vi "three_color_2D_AFM_synched.vi"() -> ()   [LabVIEW 2017]
uses:
  <vilib>/DAQmx/write.llb/DAQmx Write (Analog DBL 1Chan 1Samp).vi
  <vilib>/DAQmx/write.llb/DAQmx Write (Analog 2D DBL NChan NSamp).vi
  <vilib>/DAQmx/create/channels.llb/DAQmx Create Channel (AO-Voltage-Basic).vi
  <vilib>/DAQmx/miscellaneous.llb/DAQmx Fill In Error Info.vi
  <vilib>/DAQmx/configure/timing.llb/DAQmx Timing (Sample Clock).vi
  <vilib>/DAQmx/configure/trigger.llb/DAQmx Start Trigger (Digital Edge).vi
  <vilib>/DAQmx/write.llb/DAQmx Write (Analog 1D DBL NChan 1Samp).vi
  <resource>/objmgr/daqmx.rc
panel:
  in  "Listbox 3":i32(listbox)=3
  in  "Laser 3 (0-10v)":dbl=3.0
  out "Focal Distance (um)":dbl
  out "Diopter":dbl
  in  "ETL3 (v) [4.76V allows light passing through unaltered]":dbl(slide)=4.76 min=-10.0 max=10.0 step=0.01 scale=-10.0..10.0
  in  "Y multiplier":dbl=1.0
  in  "X multiplier":dbl=-1.0
  in  "Y (v)":dbl(slide) min=-10.0 max=10.0 step=0.01 scale=-10.0..10.0
  in  "X (v)":dbl(slide) min=-10.0 max=10.0 step=0.01 scale=-10.0..10.0
  in  "Combined Movement (v)\nEquation: X * X Multiplier + Y * Y Multiplier":dbl(slide) min=-10.0 max=10.0 step=0.01 scale=-10.0..10.0
  out "Expected AFM Frequency (HZ)":dbl
  in  "Listbox 2":i32(listbox)=3
  in  "Listbox":i32(listbox)=1
  in  "Laser 2 (0-10v)":dbl=3.0
  in  "Laser 1 (0-10v)":dbl=3.0
  in  "OFF Time(ms)":dbl=100.0
  in  "ON Time(ms)":dbl=300.0
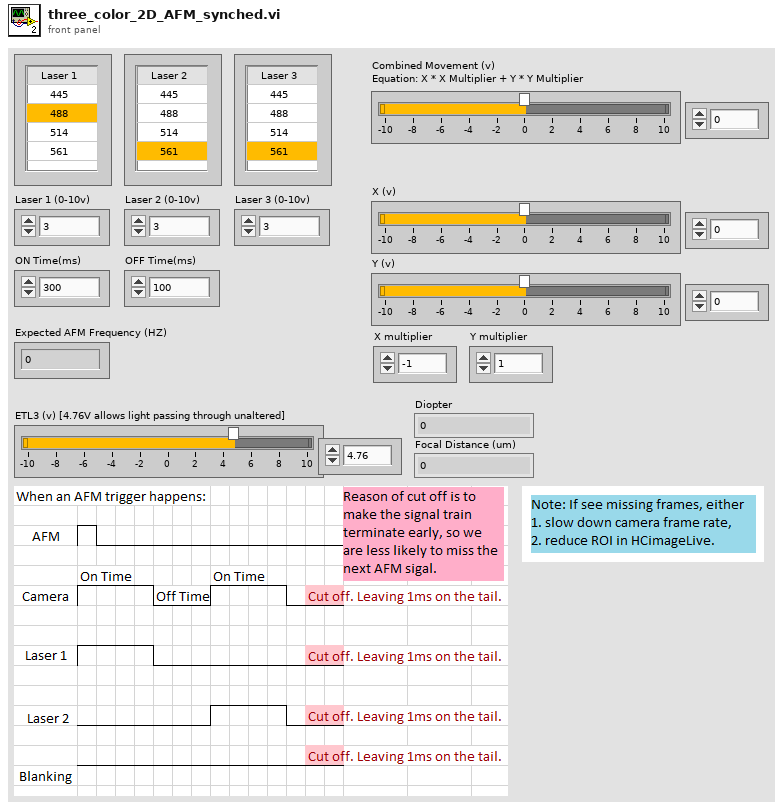
[diagram p1: front panel]
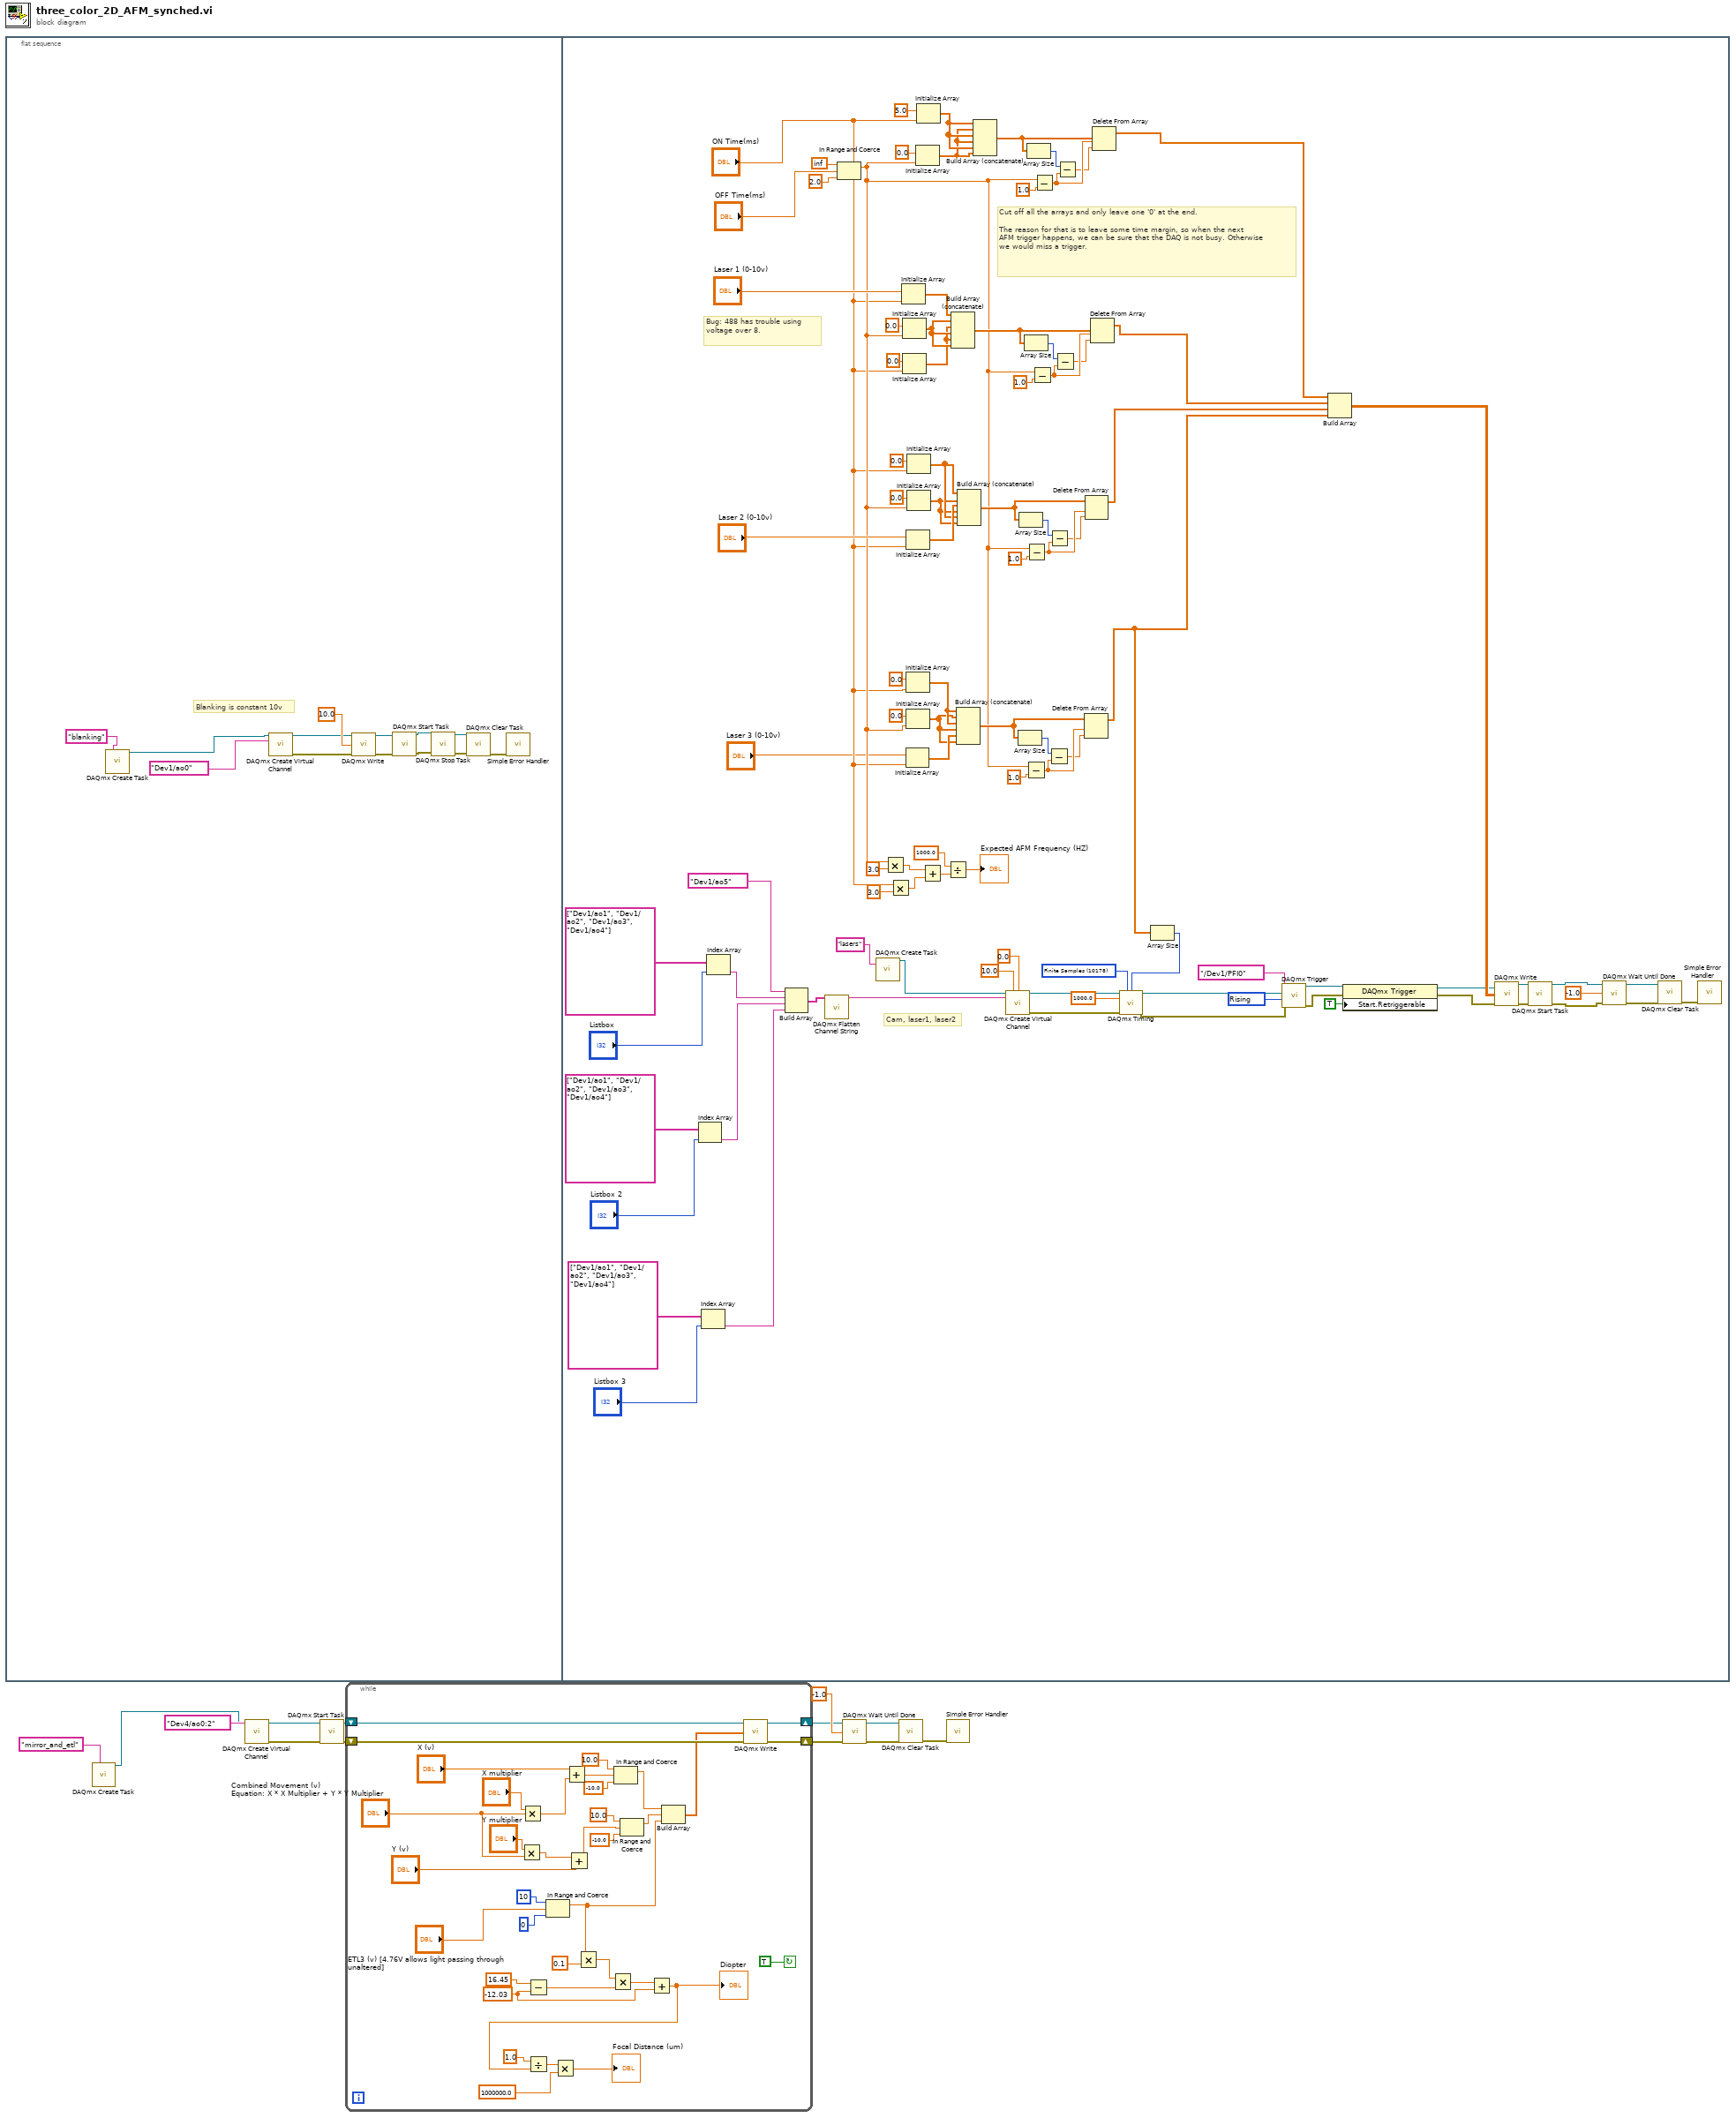
[diagram p0: block diagram]
diagram:
  n1 = flat-sequence {
    frame #0 {
      # "Blanking is constant 10v"
      n2 = call <vilib>:"DAQmx Create Task.vi"("new task name"="blanking" ("name to assign")) -> ("task out"=w16:refnum<k21>)  [unwired: 13 in, 1 out]
      n3 = call-poly <vilib>:"DAQmx Create Virtual Channel.vi"("task in"=w16, "physical channels"=tag "Dev1/ao0") -> ("task out"=w24:refnum<k21>, "error out"=w23:errorcluster)  [unwired: 12 in]
      n4 = call-poly <vilib>:"DAQmx Write.vi"("task/channels in"=w24, "data"=10.0, "error in"=w23) -> ("task out"=w22:refnum<k21>, "error out"=w21:errorcluster)  [unwired: 10 in, 1 out]
      n5 = call <vilib>:"DAQmx Start Task.vi"("task/channels in"=w22, "error in"=w21) -> ("task out"=w15:refnum<k21>, "error out"=w14:errorcluster)  [unwired: 12 in]
      n6 = call <vilib>:"DAQmx Stop Task.vi"("task/channels in"=w15, "error in"=w14) -> ("task out"=w20:refnum<k21>, "error out"=w19:errorcluster)  [unwired: 12 in]
      n7 = call <vilib>:"DAQmx Clear Task.vi"("task in"=w20, "error in"=w19) -> ("error out"=w26:errorcluster)  [unwired: 13 in]
      n8 = call <vilib>:"Simple Error Handler.vi"("error in (no error)"=w26) -> ()  [unwired: 4 in, 5 out]
    }
    frame #1 {
      w66 = 10280 items=["Rising"=10280, "Falling"=10171] ("edge")
      w62 = 10178 items=["Finite Samples"=10178, "Continuous Samples"=10123, "Hardware Timed Single Point"=12522] ("sample mode")
      # "Bug: 488 has trouble using voltage over 8."
      # "Cut off all the arrays and only leave one '0' at the end.\n\nThe reason for that is to leave some time margin, so when the next \nAFM trigger happens, we can be sure that the DAQ is not busy. Otherwise\nwe would miss a trigger."
      # "Cam, laser1, laser2"
      n9 = Index Array(array=tag[] ["Dev1/ao1", "Dev1/ao2", "Dev1/ao3", "Dev1/ao4"], index="Listbox 2") -> (element=w117:tag)
      n10 = Index Array(array=tag[] ["Dev1/ao1", "Dev1/ao2", "Dev1/ao3", "Dev1/ao4"], index="Listbox 3") -> (element=w48:tag)
      n11 = Index Array(array=tag[] ["Dev1/ao1", "Dev1/ao2", "Dev1/ao3", "Dev1/ao4"], index="Listbox") -> (element=w116:tag)
      n12 = Build Array(tag "Dev1/ao5" ("physical channels"), w116, w117, w48) -> (w118:tag[])
      n13 = call <vilib>:"DAQmx Flatten Channel String.vi"("names in"=w118) -> ("names out"=w121:string)  [unwired: 13 in, 1 out]
      n14 = In Range and Coerce(upper limit=inf, x="OFF Time(ms)", lower limit=2.0) -> (coerced(x)=w40:dbl)  [unwired: 1 out]
      n15 = call <vilib>:"DAQmx Create Task.vi"("new task name"="lasers" ("name to assign")) -> ("task out"=w123:refnum<k21>)  [unwired: 13 in, 1 out]
      n16 = Multiply(x=w40, y=3.0) -> (x*y=w106:dbl)
      n17 = Multiply(x="ON Time(ms)", y=3.0) -> (x*y=w105:dbl)
      n18 = Initialize Array("Laser 1 (0-10v)", "ON Time(ms)") -> (w80:dbl[])
      n19 = Initialize Array(0.0 ("element"), w40) -> (w33:dbl[])
      n20 = Initialize Array(0.0 ("element"), "ON Time(ms)") -> (w32:dbl[])
      n21 = Initialize Array("Laser 3 (0-10v)", "ON Time(ms)") -> (w28:dbl[])
      n22 = Initialize Array("Laser 2 (0-10v)", "ON Time(ms)") -> (w85:dbl[])
      n23 = Initialize Array(0.0 ("element"), "ON Time(ms)") -> (w29:dbl[])
      n24 = Initialize Array(0.0 ("element"), w40) -> (w27:dbl[])
      n25 = Initialize Array(0.0 ("element"), "ON Time(ms)") -> (w31:dbl[])
      n26 = Initialize Array(0.0 ("element"), w40) -> (w30:dbl[])
      n27 = Initialize Array(0.0 ("element"), w40) -> (w34:dbl[])
      n28 = Initialize Array(5.0 ("element"), "ON Time(ms)") -> (w35:dbl[])
      n29 = Add(x=w106, y=w105) -> (x+y=w107:dbl)
      n30 = Divide(x=1000.0, y=w107) -> (x/y=→"Expected AFM Frequency (HZ)":dbl)
      n31 = Build Array (concatenate)(w80, w33, w32, w33, w32, w33) -> (w84:dbl[])
      n32 = Build Array (concatenate)(w29, w27, w29, w27, w28, w27) -> (w47:dbl[])
      n33 = Build Array (concatenate)(w31, w30, w85, w30, w31, w30) -> (w89:dbl[])
      n34 = Build Array (concatenate)(w35, w34, w35, w34, w35, w34) -> (w76:dbl[])
      n35 = call-poly <vilib>:"DAQmx Create Virtual Channel.vi"("task in"=w123, "maximum value"=10.0, "minimum value"=0.0, "physical channels"=w121) -> ("task out"=w97:refnum<k21>, "error out"=w98:errorcluster)  [unwired: 10 in]
      n36 = Array Size(array=w47) -> (size(s)=w44:i32)
      n37 = Array Size(array=w89) -> (size(s)=w86:i32)
      n38 = Array Size(array=w84) -> (size(s)=w81:i32)
      n39 = Subtract(x=w40, y=1.0) -> (x-y=w46:dbl)
      n40 = Subtract(x=w40, y=1.0) -> (x-y=w88:dbl)
      n41 = Array Size(array=w76) -> (size(s)=w77:i32)
      n42 = Subtract(x=w40, y=1.0) -> (x-y=w83:dbl)
      n43 = Subtract(x=w40, y=1.0) -> (x-y=w79:dbl)
      n44 = Subtract(x=w44, y=w46) -> (x-y=w45:dbl)
      n45 = Subtract(x=w86, y=w88) -> (x-y=w87:dbl)
      n46 = Subtract(x=w81, y=w83) -> (x-y=w82:dbl)
      n47 = Subtract(x=w77, y=w79) -> (x-y=w78:dbl)
      n48 = Delete From Array(array=w47, length=w46, index=w45) -> (array with subset deleted=w36:dbl[])  [unwired: 1 out]
      n49 = Delete From Array(array=w89, length=w88, index=w87) -> (array with subset deleted=w111:dbl[])  [unwired: 1 out]
      n50 = Delete From Array(array=w84, length=w83, index=w82) -> (array with subset deleted=w109:dbl[])  [unwired: 1 out]
      n51 = Delete From Array(array=w76, length=w79, index=w78) -> (array with subset deleted=w108:dbl[])  [unwired: 1 out]
      n52 = Array Size(array=w36) -> (size(s)=w122:i32)
      n53 = call-poly <vilib>:"DAQmx Timing.vi"("task/channels in"=w97, "sample mode"=w62, "samples per channel"=w122, "rate"=1000.0, "error in"=w98) -> ("task out"=w99:refnum<k21>, "error out"=w100:errorcluster)  [unwired: 9 in]
      n54 = call-poly <vilib>:"DAQmx Trigger.vi"("task/channels in"=w99, "source"=tag "/Dev1/PFI0", "edge"=w66, "error in"=w100) -> ("task out"=w101:refnum<k21>, "error out"=w104:errorcluster)  [unwired: 10 in]
      n55 = Build Array(w108, w109, w111, w36) -> (w110:dbl[][])
      n56 = property class="DAQmx Trigger"(reference=w101, error in=w104, "Start.Retriggerable"=TRUE) -> (reference out=w102:refnum<k21>, error out=w103:errorcluster)
      n57 = call-poly <vilib>:"DAQmx Write.vi"("task/channels in"=w102, "data"=w110, "error in"=w103) -> ("task out"=w95:refnum<k21>, "error out"=w96:errorcluster)  [unwired: 10 in, 1 out]
      n58 = call <vilib>:"DAQmx Start Task.vi"("task/channels in"=w95, "error in"=w96) -> ("task out"=w94:refnum<k21>, "error out"=w93:errorcluster)  [unwired: 12 in]
      n59 = call <vilib>:"DAQmx Wait Until Done.vi"("task/channels in"=w94, "timeout (sec)"=-1.0, "error in"=w93) -> ("task out"=w91:refnum<k21>, "error out"=w92:errorcluster)  [unwired: 11 in]
      n60 = call <vilib>:"DAQmx Clear Task.vi"("task in"=w91, "error in"=w92) -> ("error out"=w90:errorcluster)  [unwired: 13 in]
      n61 = call <vilib>:"Simple Error Handler.vi"("error in (no error)"=w90) -> ()  [unwired: 4 in, 5 out]
    }
  }
  n62 = call <vilib>:"DAQmx Create Task.vi"("new task name"="mirror_and_etl" ("name to assign")) -> ("task out"=w1:refnum<k21>)  [unwired: 13 in, 1 out]
  n63 = call-poly <vilib>:"DAQmx Create Virtual Channel.vi"("task in"=w1, "physical channels"=tag "Dev4/ao0:2") -> ("task out"=w6:refnum<k21>, "error out"=w5:errorcluster)  [unwired: 12 in]
  n64 = call <vilib>:"DAQmx Start Task.vi"("task/channels in"=w6, "error in"=w5) -> ("task out"=w8:refnum<k21>, "error out"=w7:errorcluster)  [unwired: 12 in]
  n65 = while {
    shift-right: [w157] -> w3
    shift-left: w8 -> [w159]
    shift-right: [w156] -> w4
    shift-left: w7 -> [w158]
    stop <- TRUE continue-if-true
    w133 = -12.03 ("x")
    n66 = Multiply(x="Y multiplier", y="Combined Movement (v)\nEquation: X * X Multiplier + Y * Y Multiplier") -> (x*y=w144:dbl)
    n67 = Multiply(x="X multiplier", y="Combined Movement (v)\nEquation: X * X Multiplier + Y * Y Multiplier") -> (x*y=w153:dbl)
    n68 = Subtract(x=16.45 ("y"), y=w133) -> (x-y=w135:dbl)
    n69 = In Range and Coerce(upper limit=10, x="ETL3 (v) [4.76V allows light passing through unaltered]", lower limit=0) -> (coerced(x)=w132:dbl)  [unwired: 1 out]
    n70 = Add(x="X (v)", y=w153) -> (x+y=w152:dbl)
    n71 = Add(x=w144, y="Y (v)") -> (x+y=w146:dbl)
    n72 = Multiply(x=w132, y=0.1) -> (x*y=w136:dbl)
    n73 = Multiply(x=w136, y=w135) -> (x*y=w134:dbl)
    n74 = In Range and Coerce(upper limit=10.0, x=w152, lower limit=-10.0) -> (coerced(x)=w149:dbl)  [unwired: 1 out]
    n75 = In Range and Coerce(upper limit=10.0, x=w146, lower limit=-10.0) -> (coerced(x)=w145:dbl)  [unwired: 1 out]
    n76 = Add(x=w134, y=w133) -> (x+y=w127:dbl)
    "Diopter" <- w127
    n77 = Divide(x=1.0, y=w127) -> (x/y=w142:dbl)
    n78 = Multiply(x=w142, y=1000000.0) -> (x*y=→"Focal Distance (um)":dbl)
    n79 = Build Array(w149, w145, w132) -> (w155:dbl[])
    n80 = call-poly <vilib>:"DAQmx Write.vi"("task/channels in"=w159, "data"=w155, "error in"=w158) -> ("task out"=w157:refnum<k21>, "error out"=w156:errorcluster)  [unwired: 10 in, 1 out]
  }
  n81 = call <vilib>:"DAQmx Wait Until Done.vi"("task/channels in"=w3, "timeout (sec)"=-1.0, "error in"=w4) -> ("task out"=w12:refnum<k21>, "error out"=w11:errorcluster)  [unwired: 11 in]
  n82 = call <vilib>:"DAQmx Clear Task.vi"("task in"=w12, "error in"=w11) -> ("error out"=w13:errorcluster)  [unwired: 13 in]
  n83 = call <vilib>:"Simple Error Handler.vi"("error in (no error)"=w13) -> ()  [unwired: 4 in, 5 out]
